vi "getBackNode.vi"(8 "error in (no error)":errorcluster, 11 "LLNode in":refnum<class "LLNode.lvclass">) -> (0 "error out":errorcluster, 2 "BackNode":refnum<data-value>, 3 "LLNode out":refnum<class "LLNode.lvclass">)   [LabVIEW 2009, in "LLNode.lvclass"]
uses:
  LLNode.lvclass
  DataObj/DataObj.lvclass
  Node/Node.lvclass
  LLNode.lvclass/LLNode.ctl
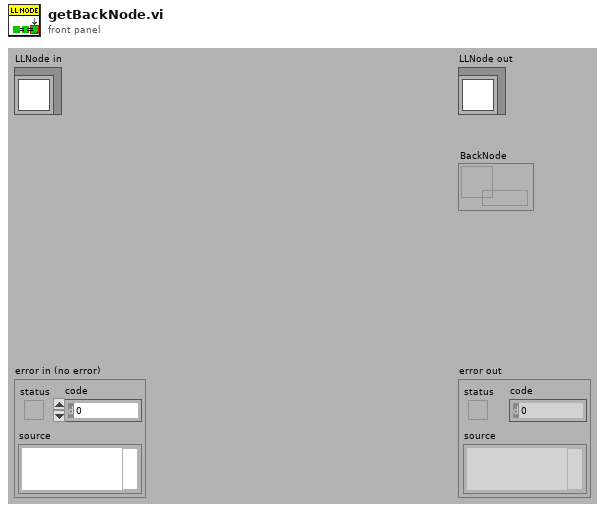
[diagram p1: front panel]
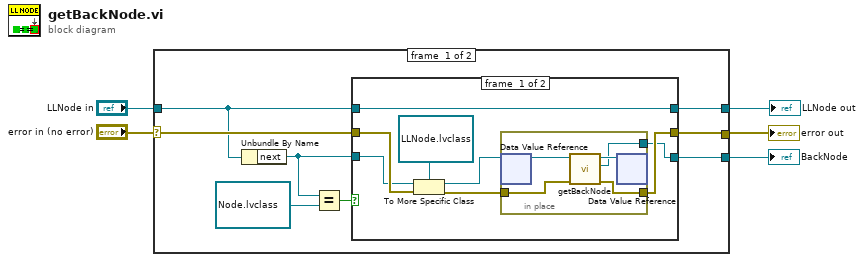
[diagram p0: block diagram]
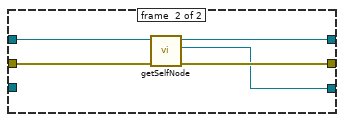
[diagram p2: hidden frame]
diagram:
  n1 = case shown="No Error" "error in (no error)" {
    selector: "error in (no error)" -> [w11 w33]
    tunnel: [w9 w33] -> w4
    tunnel: [w6 w32] -> w2
    tunnel: "LLNode in" -> [w7 w32]
    tunnel: [w10 _] -> w1
    frame #0 {
      n2 = Unbundle By Name(w7) -> ("next"=w8:refnum<data-value>)
      n3 = Equal?(x=w8, y=refnum<data-value> refnum) -> (x = y?=w12:bool)
      n4 = case shown="False" w12 {
        tunnel: w11 -> [w20 w31]
        tunnel: [w17 w30] -> w9
        tunnel: [w16 w29] -> w10
        tunnel: w8 -> [w18 _]
        tunnel: w7 -> [w21 w28]
        tunnel: [w21 w27] -> w6
        frame #0 {
          n5 = To More Specific Class(target class=refnum<data-value> refnum ("data value reference"), reference=w18, error in=w20) -> (specific class reference=w15:refnum<data-value>, error out=w19:errorcluster)
          n6 = in-place {
            in-place-border: w19 -> [w26]
            in-place-border: [w23] -> w17
            in-place-border: [w22] -> w16
            n7 = in-place-dvr #1(w15) -> (w24:refnum<class "LLNode.lvclass">)  [unwired: 1 out]
            n8 = call "getBackNode.vi"("error in (no error)"=w26, "LLNode in"=w24) -> ("error out"=w23:errorcluster, "BackNode"=w22:refnum<data-value>, "LLNode out"=w25:refnum<class "LLNode.lvclass">)  [unwired: 7 in]
            n9 = in-place-dvr #1(w25) -> ()  [unwired: 2 out]
          }
        }
        frame #1 {
          n10 = call "getSelfNode.vi"("error in (no error)"=w31, "Node in"=w28) -> ("error out"=w30:errorcluster, "selfNode"=w29:refnum<data-value>, "Node out"=w27:refnum<class "LLNode.lvclass">)  [unwired: 7 in]
        }
      }
    }
    frame #1 {
    }
  }
  "error out" <- w4
  "LLNode out" <- w2
  "BackNode" <- w1
